vi "MergeDiffPngFiles.vi"(9 "Before = F | After = T?":bool, 10 "Diff PNG Files":path[](array[path])) -> ()   [LabVIEW 2020]
uses:
  4bd7a358-025b-436a-b08a-e2c5914ece35.vi
  6fabf7ea-5db0-41f0-8f7d-caee261b24fd.vi
  <vilib>/numeric/Random Number (Range) I64.vi
  <vilib>/numeric/sub_Random U32.vi
  <vilib>/Comparison/Equal/Equal Functor/Equal Functor.lvclass
panel:
  out "colors":u32[](array[colorbox])
  out "clean picture":picture
  out "size(s)":i32[](array[numeric])
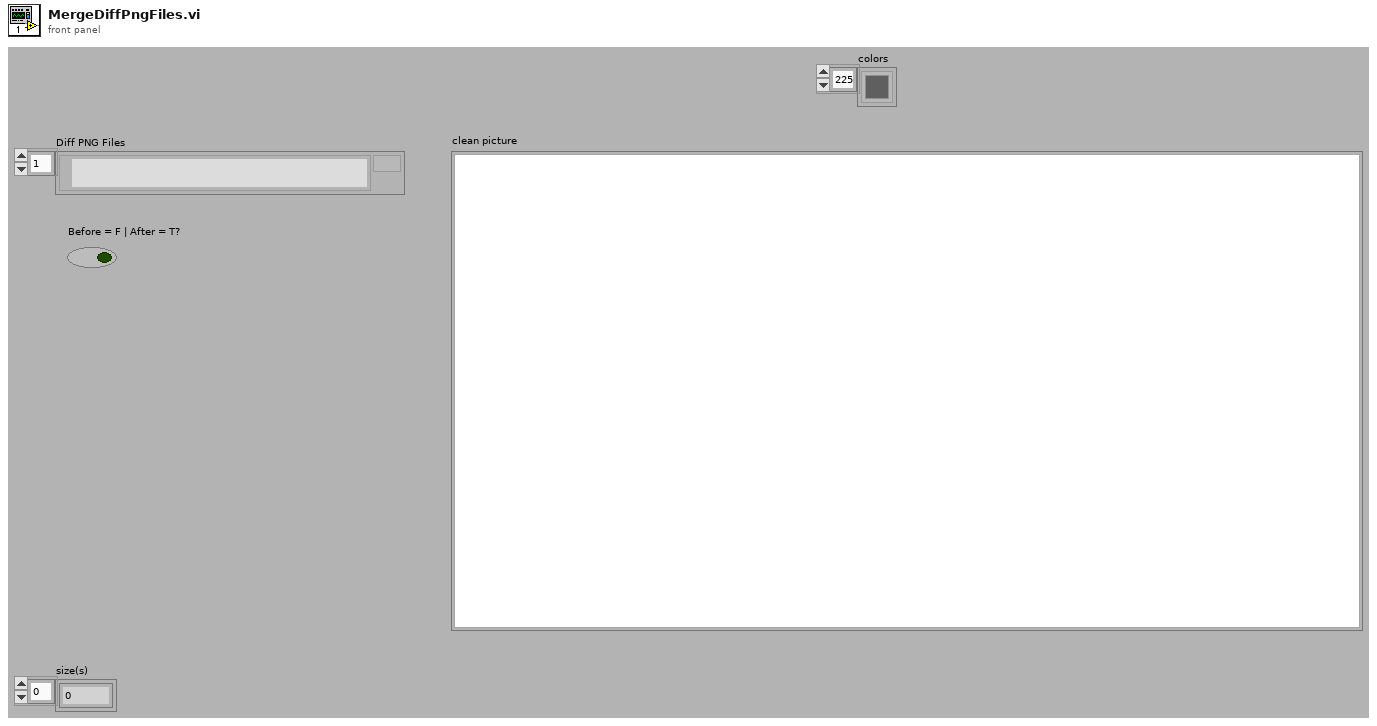
[diagram p1: front panel]
types:
  T1 = typedef "imagedata.ctl" = cluster{"image type":i32, "image depth":i32, "image":u8[], "mask":u8[], "colors":u32[], "Rectangle":cluster{"left":i16, "top":i16, "right":i16, "bottom":i16}}
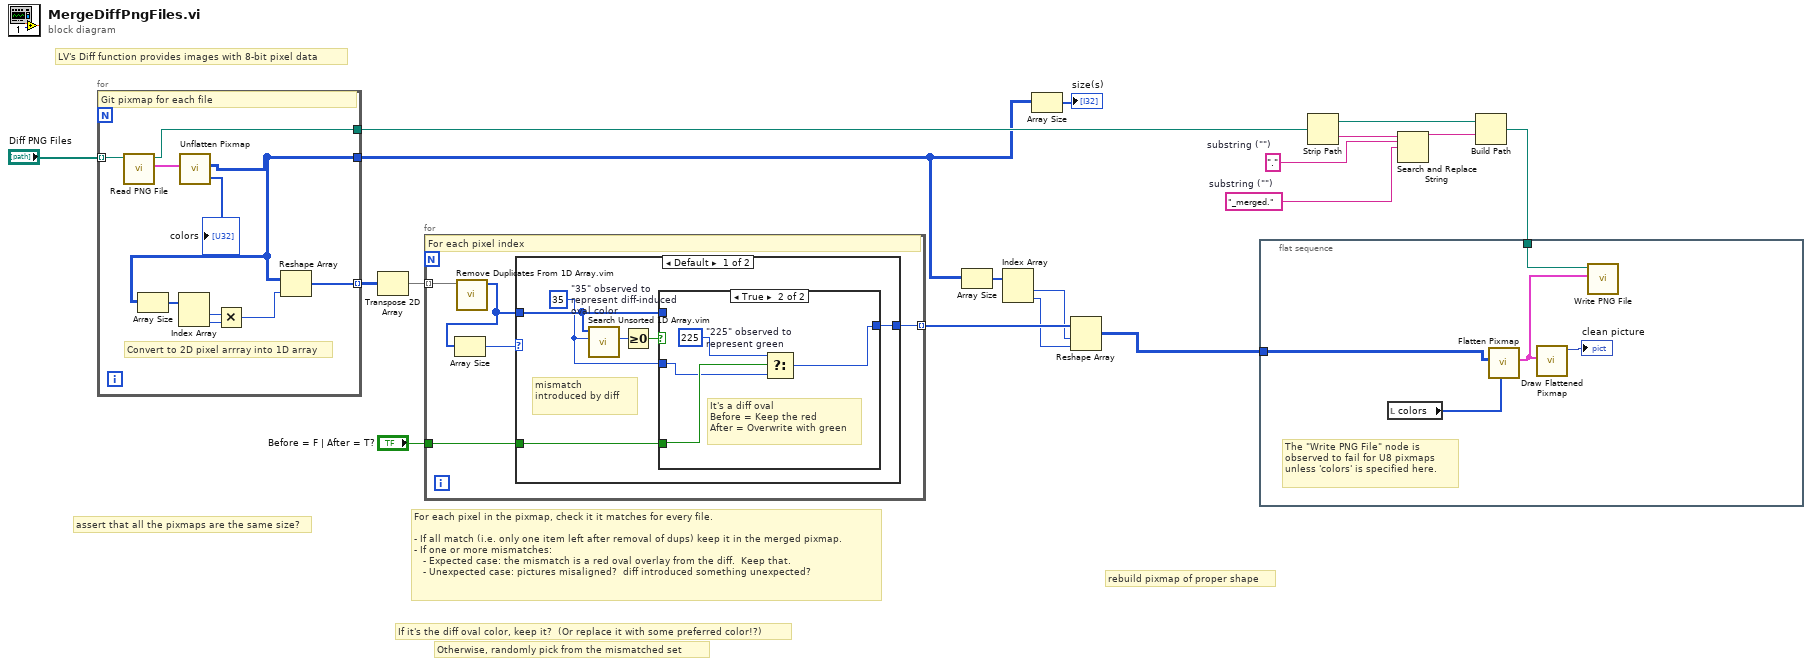
[diagram p0: block diagram]
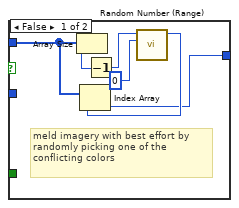
[diagram p2: hidden frame]
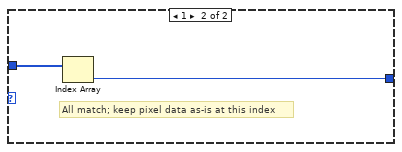
[diagram p3: hidden frame]
diagram:
  w13 = "_merged."  # substring ("")
  w14 = "."  # substring ("")
  # "If it's the diff oval color, keep it?  (Or replace it with some preferred color!?)"
  # "Otherwise, randomly pick from the mismatched set"
  # "LV's Diff function provides images with 8-bit pixel data"
  # "rebuild pixmap of proper shape"
  # "assert that all the pixmaps are the same size?"
  # "For each pixel in the pixmap, check it it matches for every file.\n\n- If all match (i.e. only one item left after removal of dups) keep it in the merged pixmap.\n- If one or more mismatches:\n   - Expected case: the mismatch is a red oval overlay from the diff.  Keep that.\n   - Unexpected case: pictures misaligned?  diff introduced something unexpected?"
  n1 = for {
    tunnel: [w20] -> w5
    tunnel: [w27] -> w17
    tunnel: "Diff PNG Files" -> [w26] mode=indexing
    tunnel: [w25] -> w9 mode=indexing
    # "Convert to 2D pixel arrray into 1D array"
    # "Git pixmap for each file"
    n2 = call <vilib>:"Read PNG File.vi"("path to PNG file"=w26) -> ("image data"=w28:T1, "path"=w27:path)  [unwired: 8 in, 1 out]
    n3 = call <vilib>:"Unflatten Pixmap.vi"("image data"=w28) -> ("8-bit pixmap"=w20:u8[][], "colors"=→"colors":u32[])  [unwired: 4 in, 5 out]
    n4 = Array Size(array=w20) -> (size(s)=w24:i32[])
    n5 = Index Array(array=w24) -> (element #1=w22:i32, element #2=w23:i32)  [unwired: 2 in]
    n6 = Multiply(x=w22, y=w23) -> (x*y=w21:i32)
    n7 = Reshape Array(w20, w21) -> (w25:u8[])
  }
  n8 = Transpose 2D Array(2D array=w9) -> (transposed array=w8:u8[][])
  n9 = for {
    tunnel: w8 -> [w33] mode=indexing
    tunnel: [w30] -> w7 mode=indexing
    tunnel: "Before = F | After = T?" -> [w29]
    # "For each pixel index"
    n10 = call "Remove Duplicates From 1D Array.vim"("array"=w33) -> ("array with duplicates removed"=w31:u8[])  [unwired: 10 in]
    n11 = Array Size(array=w31) -> (size(s)=w32:i32)
    n12 = case shown="Default" w32 {
      tunnel: w31 -> [w38 w51]
      tunnel: [w39 w50] -> w30
      tunnel: w29 -> [w34 _]
      frame Default {
        w35 = u8 35  # "35" observed to represent diff-induced oval color
        # "mismatch introduced by diff"
        n13 = call "Search Unsorted 1D Array.vim"("element"=w35, "unsorted 1D array"=w38) -> ("index of element"=w37:i32)  [unwired: 9 in]
        n14 = Greater Or Equal To 0?(x=w37) -> (x >= 0?=w36:bool)
        n15 = case shown="True" w36 {
          tunnel: [w43 w46] -> w39
          tunnel: w38 -> [w40 _]
          tunnel: w35 -> [_ w48]
          tunnel: w34 -> [_ w49]
          frame False {
            # "meld imagery with best effort by randomly picking one of the conflicting colors"
            n16 = Array Size(array=w40) -> (size(s)=w45:i32)
            n17 = Decrement(x=w45) -> (x-1=w42:i32)
            n18 = call-poly <vilib>:"Random Number (Range).vi"("lower bound (-100)"=i64 0, "upper bound (100)"=w42) -> ("number"=w44:i64)  [unwired: 9 in]
            n19 = Index Array(array=w40, index=w44) -> (element=w43:u8)
          }
          frame True {
            w47 = u8 225  # "225" observed to represent green
            # "It's a diff oval\nBefore = Keep the red\nAfter = Overwrite with green"
            n20 = Select(t=w47, s=w49, f=w48) -> (s? t:f=w46:u8)
          }
        }
      }
      frame 1 {
        # "All match; keep pixel data as-is at this index"
        n21 = Index Array(array=w51) -> (element=w50:u8)  [unwired: 1 in]
      }
    }
  }
  n22 = Array Size(array=w5) -> (size(s)=w6:i32[])
  n23 = Index Array(array=w6) -> (element #1=w4:i32, element #2=w3:i32)  [unwired: 2 in]
  n24 = Array Size(array=w5) -> (size(s)=→"size(s)":i32[])
  n25 = Reshape Array(w7, w4, w3) -> (w2:u8[][])
  n26 = flat-sequence {
    tunnel: w11 -> [w54]
    tunnel: w2 -> [w53]
    frame #0 {
      # "The \"Write PNG File\" node is observed to fail for U8 pixmaps unless 'colors' is specified here."
      n27 = local read "colors"() -> (w52:u32[])
      n28 = call <vilib>:"Flatten Pixmap.vi"("colors"=w52, "8-bit pixmap"=w53) -> ("image data"=w55:T1)  [unwired: 9 in]
      n29 = call <vilib>:"Draw Flattened Pixmap.vi"("image data"=w55) -> ("new picture"=→"clean picture":picture)  [unwired: 8 in]
      n30 = call <vilib>:"Write PNG File.vi"("image data"=w55, "path to PNG file"=w54) -> ()  [unwired: 8 in, 2 out]
    }
  }
  n31 = Strip Path(path=w17) -> (stripped path=w16:path, name=w15:string)
  n32 = Search and Replace String(input string=w15, search string=w14, replace string=w13) -> (result string=w12:string)  [unwired: 5 in, 3 out]
  n33 = Build Path(base path=w16, name or relative path=w12) -> (appended path=w11:path)
